vi "IMAQ FPGA Camera Link Acquisition State Machine.vi"(8 "Enables":T2, 9 "Cancel Acq":bool, 10 "Acquire":bool, 11 "Acquisition Settings":T3) -> (0 "Output Valid":bool, 1 "Frame Valid":bool, 2 "Line Valid":bool, 3 "Acquisition Status":T1, 5 "Reset":bool)   [LabVIEW 2020]
doc: "The Acquisition State Machine VI monitors the Camera Link enable signals to determine when pixel data should be captured and when it should be ignored, as indicated by the <B>Output Valid</B>, <B>Frame Valid</B>, and <B>Line Valid</B> outputs. The VI supports finite and continuous acquisitions for both area and line scan cameras. This VI is intended to run within a single-cycle timed loop.\n\nNote that the outputs are delayed by two clock cycles relative to the inputs. Also, this VI does not support cameras that change FVAL while LVAL is asserted. However, FVAL and LVAL are allowed to change at the same time. Open the VI for more documentation."
uses:
  <vilib>/visionFPGA/Basics/Camera Link Acquisition/Controls/IMAQ FPGA Camera Link Acquisition State.ctl
panel:
  # "Refer to the Context Help for a\ndescription of the controls and\nindicators of this VI."
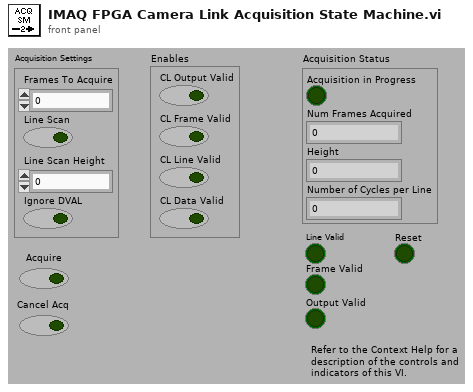
[diagram p1: front panel]
types:
  T1 = cluster{"Acquisition in Progress":bool, "Num Frames Acquired":u32, "Height":u32, "Number of Cycles per Line":u32}
  T2 = cluster{"CL Output Valid":bool, "CL Frame Valid":bool, "CL Line Valid":bool, "CL Data Valid":bool}
  T3 = cluster{"Frames To Acquire":u32, "Line Scan":bool, "Line Scan Height":u32, "Ignore DVAL":bool}
  T4 = typedef "IMAQ FPGA Camera Link Acquisition State.ctl" = enum16{"Idle", "WaitForBlanking", "WaitForStartOfFrame", "WaitForEndOfFrame", "WaitForLastTransition"}
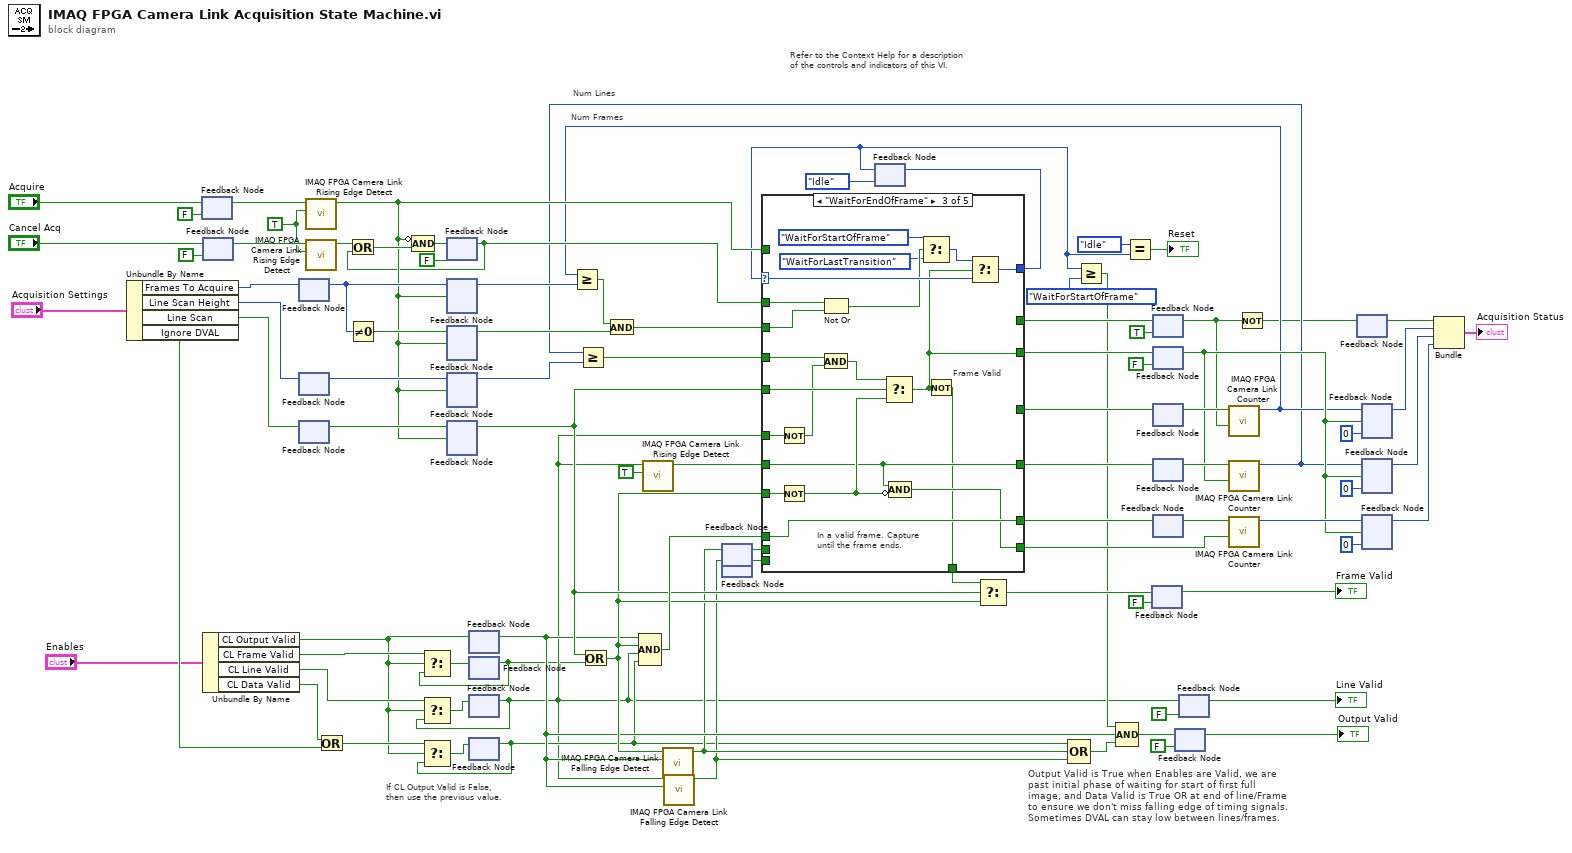
[diagram p0: block diagram]
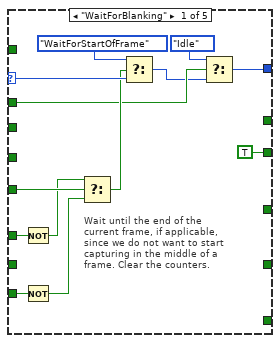
[diagram p2: hidden frame]
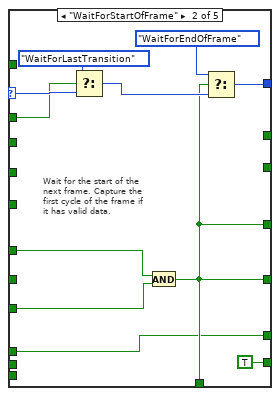
[diagram p3: hidden frame]
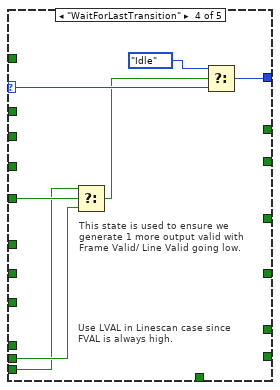
[diagram p4: hidden frame]
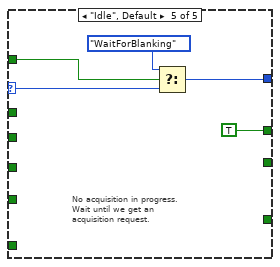
[diagram p5: hidden frame]
diagram:
  w31 = TRUE ("Input Valid")
  # "If CL Output Valid is False,\nthen use the previous value."
  # "Num Lines"
  # "Num Frames"
  # "Output Valid is True when Enables are Valid, we are past initial phase of waiting for start of first full image, and Data Valid is True OR at end of line/Frame to ensure we don't miss falling edge of timing signals. Sometimes DVAL can stay low between lines/frames."
  # "Refer to the Context Help for a description\nof the controls and indicators of this VI."
  n1 = Unbundle By Name("Acquisition Settings") -> ("Frames To Acquire"=w43:u32, "Line Scan Height"=w42:u32, "Line Scan"=w41:bool, "Ignore DVAL"=w40:bool)
  n2 = feedback #1(FALSE ("Acquire")) -> (w37:bool)
  n3 = feedback-in #1("Acquire") -> ()
  n4 = feedback #2(FALSE ("Cancel Acq")) -> (w32:bool)
  n5 = feedback-in #2("Cancel Acq") -> ()
  n6 = Unbundle By Name("Enables") -> ("CL Output Valid"=w1:bool, "CL Frame Valid"=w4:bool, "CL Line Valid"=w7:bool, "CL Data Valid"=w38:bool)
  n7 = feedback #3() -> (w79:u32)  [unwired: 1 in]
  n8 = feedback-in #3(w43) -> ()
  n9 = feedback #4() -> (w72:u32)  [unwired: 1 in]
  n10 = feedback-in #4(w42) -> ()
  n11 = feedback #5() -> (w71:bool)  [unwired: 1 in]
  n12 = feedback-in #5(w41) -> ()
  n13 = call <vilib>:"IMAQ FPGA Camera Link Rising Edge Detect.vi"("Input Valid"=w31, "Input"=w37) -> ("Rising Edge"=w36:bool)  [unwired: 9 in]
  n14 = call <vilib>:"IMAQ FPGA Camera Link Rising Edge Detect.vi"("Input Valid"=w31, "Input"=w32) -> ("Rising Edge"=w30:bool)  [unwired: 9 in]
  n15 = Or(x=w38, y=w40) -> (x .or. y?=w10:bool)
  n16 = Not Equal To 0?(x=w79) -> (x != 0?=w88:bool)
  n17 = feedback #6(FALSE) -> (w33:bool)
  n18 = Or(x=w30, y=w33) -> (x .or. y?=w75:bool)
  n19 = Compound Arithmetic op=AND(invert w36, w75) -> (w74:bool)
  n20 = feedback-in #6(w74) -> ()
  n21 = feedback #7() -> (w85:u32)  [unwired: 1 in]
  n22 = feedback-in #7(w79, w36) -> ()
  n23 = feedback #8() -> (w86:bool)  [unwired: 1 in]
  n24 = feedback-in #8(w88, w36) -> ()
  n25 = feedback #9() -> (w70:u32)  [unwired: 1 in]
  n26 = feedback-in #9(w72, w36) -> ()
  n27 = feedback #10() -> (w57:bool)  [unwired: 1 in]
  n28 = feedback-in #10(w71, w36) -> ()
  n29 = feedback #11() -> (w25:bool)  [unwired: 1 in]
  n30 = feedback-in #11(w1) -> ()
  n31 = feedback #12() -> (w2:bool)  [unwired: 1 in]
  n32 = Select(t=w4, s=w1, f=w2) -> (s? t:f=w3:bool)
  n33 = feedback-in #12(w3) -> ()
  n34 = feedback #13() -> (w6:bool)  [unwired: 1 in]
  n35 = Select(t=w7, s=w1, f=w6) -> (s? t:f=w5:bool)
  n36 = feedback-in #13(w5) -> ()
  n37 = feedback #14() -> (w8:bool)  [unwired: 1 in]
  n38 = Select(t=w10, s=w1, f=w8) -> (s? t:f=w9:bool)
  n39 = feedback-in #14(w9) -> ()
  n40 = Or(x=w57, y=w2) -> (x .or. y?=w48:bool)
  n41 = Compound Arithmetic op=AND(w25, w48, w6, w8) -> (w76:bool)
  n42 = call <vilib>:"IMAQ FPGA Camera Link Rising Edge Detect.vi"("Input Valid"=TRUE, "Input"=w6) -> ("Rising Edge"=w73:bool)  [unwired: 9 in]
  n43 = call <vilib>:"IMAQ FPGA Camera Link Falling Edge Detect.vi"("Input Valid"=w25, "Input"=w48) -> ("Falling Edge"=w24:bool)  [unwired: 9 in]
  n44 = call <vilib>:"IMAQ FPGA Camera Link Falling Edge Detect.vi"("Input Valid"=w25, "Input"=w6) -> ("Falling Edge"=w22:bool)  [unwired: 9 in]
  n45 = feedback #15() -> (w23:bool)  [unwired: 1 in]
  n46 = feedback-in #15(w24) -> ()
  n47 = feedback #16() -> (w21:bool)  [unwired: 1 in]
  n48 = feedback-in #16(w22) -> ()
  n49 = feedback #17(IMAQ_FPGA_Camera_Link_Acquisition_State."Idle" ("Enum")) -> (w26:T4)
  n50 = Compound Arithmetic op=OR(w8, w24, w22) -> (w49:bool)
  n51 = Greater Or Equal?(x=w26, y=IMAQ_FPGA_Camera_Link_Acquisition_State."WaitForStartOfFrame") -> (x >= y?=w50:bool)
  n52 = Compound Arithmetic op=AND(w50, w25, w49) -> (w51:bool)
  n53 = Equal?(x=IMAQ_FPGA_Camera_Link_Acquisition_State."Idle", y=w26) -> (x = y?=→"Reset":bool)
  n54 = feedback #18(FALSE) -> (→"Frame Valid":bool)
  n55 = feedback #19(TRUE) -> (w17:bool)
  n56 = feedback #20(FALSE) -> (w62:bool)
  n57 = feedback #21() -> (w90:bool)  [unwired: 1 in]
  n58 = feedback #22() -> (w91:bool)  [unwired: 1 in]
  n59 = feedback #23() -> (w82:bool)  [unwired: 1 in]
  n60 = feedback #24(FALSE) -> (→"Output Valid":bool)
  n61 = feedback-in #24(w51) -> ()
  n62 = feedback-in #25(w6) -> ()
  n63 = feedback #25(FALSE) -> (→"Line Valid":bool)
  n64 = call <vilib>:"IMAQ FPGA Camera Link Counter.vi"("Restart?"=w17, "Increment?"=w90) -> ("Count"=w20:u32)  [unwired: 9 in]
  n65 = Greater Or Equal?(x=w20, y=w85) -> (x >= y?=w87:bool)
  n66 = And(x=w87, y=w86) -> (x .and. y?=w46:bool)
  n67 = call <vilib>:"IMAQ FPGA Camera Link Counter.vi"("Restart?"=w62, "Increment?"=w91) -> ("Count"=w19:u32)  [unwired: 9 in]
  n68 = Greater Or Equal?(x=w19, y=w70) -> (x >= y?=w61:bool)
  n69 = case shown="\"WaitForEndOfFrame\"" w26 {
    selector: w26 -> [w105 w116 w135 w143 w147]
    tunnel: [w98 w113 w136 w142 w148] -> w27
    tunnel: w36 -> [_ _ _ _ w146]
    tunnel: w48 -> [w103 w110 w125 _ _]
    tunnel: [_ w109 w122 _ _] -> w92
    tunnel: [_ w109 _ _ _] -> w89
    tunnel: [TRUE _ w121 _ _] -> w64
    tunnel: w46 -> [_ _ w127 _ _]
    tunnel: [_ _ _ _ TRUE] -> w84
    tunnel: [_ w108 w134 _ _] -> w81
    tunnel: w76 -> [_ w108 w134 _ _]
    tunnel: [_ TRUE w124 _ _] -> w80
    tunnel: w73 -> [_ _ w122 _ _]
    tunnel: w61 -> [_ _ w129 _ _]
    tunnel: w57 -> [w104 _ w132 w140 _]
    tunnel: w33 -> [w100 w112 w128 _ _]
    tunnel: w6 -> [w97 w111 w119 _ _]
    tunnel: [_ w109 w120 _ _] -> w56
    tunnel: w23 -> [_ _ _ w138 _]
    tunnel: w21 -> [_ _ _ w137 _]
    frame "WaitForBlanking" {
      # "Wait until the end of the\ncurrent frame, if applicable,\nsince we do not want to start capturing in the middle of a frame. Clear the counters."
      n70 = Not(x=w97) -> (.not. x?=w96:bool)
      n71 = Not(x=w103) -> (.not. x?=w101:bool)
      n72 = Select(t=w96, s=w104, f=w101) -> (s? t:f=w102:bool)
      n73 = Select(t=IMAQ_FPGA_Camera_Link_Acquisition_State."WaitForStartOfFrame" ("Enum"), s=w102, f=w105) -> (s? t:f=w99:T4)
      n74 = Select(t=IMAQ_FPGA_Camera_Link_Acquisition_State."Idle" ("Enum"), s=w100, f=w99) -> (s? t:f=w98:T4)
    }
    frame "WaitForStartOfFrame" {
      # "Wait for the start of the\nnext frame. Capture the\nfirst cycle of the frame if\nit has valid data."
      n75 = Select(t=IMAQ_FPGA_Camera_Link_Acquisition_State."WaitForLastTransition" ("Enum"), s=w112, f=w116) -> (s? t:f=w114:T4)
      n76 = And(x=w111, y=w110) -> (x .and. y?=w109:bool)
      n77 = Select(t=IMAQ_FPGA_Camera_Link_Acquisition_State."WaitForEndOfFrame" ("Enum"), s=w109, f=w114) -> (s? t:f=w113:T4)
    }
    frame "WaitForEndOfFrame" {
      # "Frame Valid"
      # "In a valid frame. Capture\nuntil the frame ends."
      n78 = Not(x=w119) -> (.not. x?=w131:bool)
      n79 = Not(x=w125) -> (.not. x?=w123:bool)
      n80 = Not Or(1:w127, 2:w128) -> (0:w126:bool)
      n81 = And(x=w129, y=w131) -> (x .and. y?=w130:bool)
      n82 = Select(t=w130, s=w132, f=w123) -> (s? t:f=w121:bool)
      n83 = Compound Arithmetic op=AND(w122, invert w123) -> (w124:bool)
      n84 = Select(t=IMAQ_FPGA_Camera_Link_Acquisition_State."WaitForStartOfFrame" ("Enum"), s=w126, f=IMAQ_FPGA_Camera_Link_Acquisition_State."WaitForLastTransition") -> (s? t:f=w133:T4)
      n85 = Not(x=w121) -> (.not. x?=w120:bool)
      n86 = Select(t=w133, s=w121, f=w135) -> (s? t:f=w136:T4)
    }
    frame "WaitForLastTransition" {
      # "This state is used to ensure we generate 1 more output valid with Frame Valid/ Line Valid going low."
      # "Use LVAL in Linescan case since FVAL is always high."
      n87 = Select(t=w137, s=w140, f=w138) -> (s? t:f=w139:bool)
      n88 = Select(t=IMAQ_FPGA_Camera_Link_Acquisition_State."Idle", s=w139, f=w143) -> (s? t:f=w142:T4)
    }
    frame "Idle", Default {
      # "No acquisition in progress.\nWait until we get an\nacquisition request."
      n89 = Select(t=IMAQ_FPGA_Camera_Link_Acquisition_State."WaitForBlanking", s=w146, f=w147) -> (s? t:f=w148:T4)
    }
  }
  n90 = feedback-in #17(w27) -> ()
  n91 = Select(t=w56, s=w57, f=w48) -> (s? t:f=w55:bool)
  n92 = feedback-in #18(w55) -> ()
  n93 = feedback-in #19(w84) -> ()
  n94 = feedback-in #20(w64) -> ()
  n95 = feedback-in #21(w89) -> ()
  n96 = feedback-in #22(w92) -> ()
  n97 = feedback-in #23(w81) -> ()
  n98 = call <vilib>:"IMAQ FPGA Camera Link Counter.vi"("Restart?"=w80, "Increment?"=w82) -> ("Count"=w83:u32)  [unwired: 9 in]
  n99 = Not(x=w17) -> (.not. x?=w16:bool)
  n100 = feedback #26() -> (w15:bool)  [unwired: 1 in]
  n101 = feedback-in #26(w16) -> ()
  n102 = feedback #27(u32 0 ("Count")) -> (w14:u32)
  n103 = feedback-in #27(w20, w62) -> ()
  n104 = feedback #28(u32 0) -> (w13:u32)
  n105 = feedback-in #28(w19, w62) -> ()
  n106 = feedback #29(u32 0 ("Count")) -> (w12:u32)
  n107 = feedback-in #29(w83, w62) -> ()
  n108 = Bundle(w15, "Count"=w14, w13, "Count"=w12) -> (→"Acquisition Status":cluster{bool, "Count":u32, u32, "Count":u32})  [unwired: 1 in]
